vi "Read Resource Name.vi"(8 "error in (no error)":errorcluster, 11 "NICal5501 in":refnum<class "Cal Standard.lvclass">) -> (0 "error out":errorcluster, 2 "Resource Name":refnum<k15>, 3 "NICal5501 out":refnum<class "Cal Standard.lvclass">)   [LabVIEW 2023, in "NI Cal-5501 Cal Standard.lvlib" / "Cal Standard.lvclass"]
uses:
  Cal Standard.lvclass
  Cal Standard.lvclass/Cal Standard.ctl
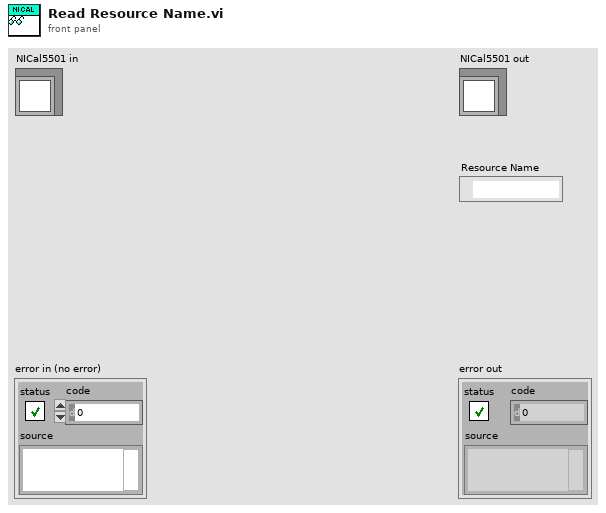
[diagram p1: front panel]
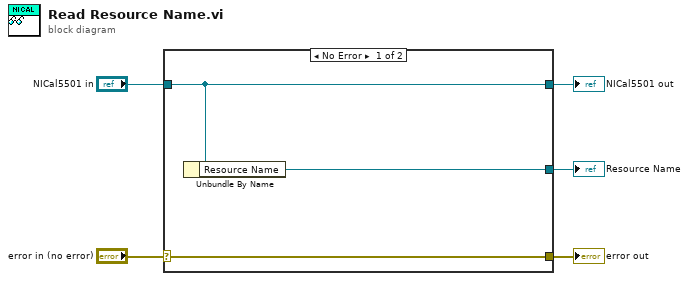
[diagram p0: block diagram]
diagram:
  n1 = case shown="No Error" "error in (no error)" {
    selector: "error in (no error)" -> [w8 w9]
    tunnel: [w8 w9] -> w4
    tunnel: [w7 w10] -> w2
    tunnel: "NICal5501 in" -> [w7 w10]
    tunnel: [w6 _] -> w1
    frame No Error {
      n2 = Unbundle By Name(w7) -> ("Resource Name"=w6:refnum<k15>)
    }
    frame Error {
    }
  }
  "error out" <- w4
  "NICal5501 out" <- w2
  "Resource Name" <- w1
